vi "Write Cells pos.vi"(8 "error in (no error)":errorcluster, 10 "Cells pos":dbl[](array[numeric]), 11 "Control-Client in":refnum<class "Control-Client.lvclass">) -> (0 "error out":errorcluster, 3 "Control-Client out":refnum<class "Control-Client.lvclass">)   [LabVIEW 2019, in "Control-Client.lvclass"]
uses:
  Control-Client.lvclass
  Control-Client.lvclass/Control-Client.ctl
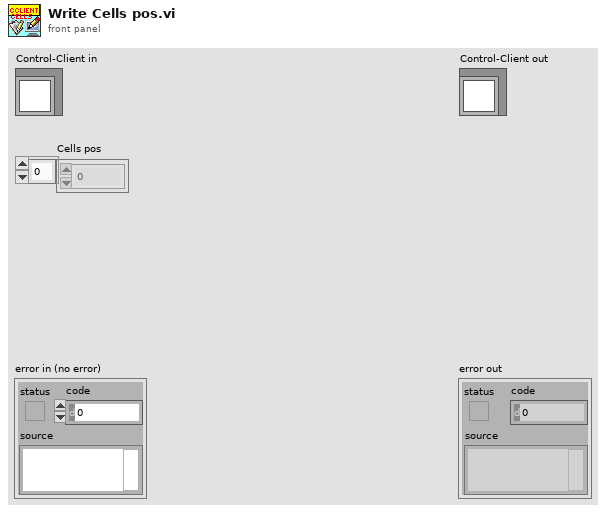
[diagram p1: front panel]
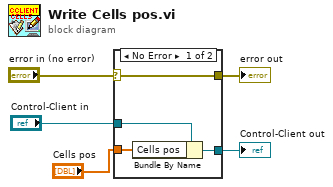
[diagram p0: block diagram]
diagram:
  n1 = case shown="No Error" "error in (no error)" {
    selector: "error in (no error)" -> [w9 w10]
    tunnel: [w9 w10] -> w4
    tunnel: [w7 w11] -> w2
    tunnel: "Control-Client in" -> [w8 w11]
    tunnel: "Cells pos" -> [w6 _]
    frame No Error {
      n2 = Bundle By Name(cluster=w8, "Cells pos"=w6) -> (w7:refnum<class "Control-Client.lvclass">)
    }
    frame Error {
    }
  }
  "error out" <- w4
  "Control-Client out" <- w2
